vi "serial-read-subVi-SAFEish.vi"(8 "error in":errorcluster, 10 "state":string="init", 11 "VISA resource name":refnum<visa-resource-name>="COM22") -> (0 "error out":errorcluster, 1 "read buffer out":string, 2 "all-sensor-data":T4 {"CD4"."CO2 (ppm)" format="%.2f"; "CD3"."CO2 (ppm)" format="%.2f"; "RHT4"."Humidity (%)" format="%.2f"; "RHT4"."Temp (degC)" format="%.2f"; "RHT5"."Humidity (%)" format="%.2f"; "RHT5"."Temp (degC)" format="%.2f"; "CD2"."Humidity (%)" format="%.2f"; "CD2"."Temp (degC)" format="%.2f"; "CD2"."CO2 (ppm)" format="%.2f"; "RHT3"."Humidity (%)" format="%.2f"; "RHT3"."Temp (degC)" format="%.2f"; "CD6"."CO2 (ppm)" format="%.2f"; "RHT6"."Humidity (%)" format="%.2f"; "RHT6"."Temp (degC)" format="%.2f"; "CD5"."CO2 (ppm)" format="%.2f"; "CD1"."Humidity (%)" format="%.2f"; "CD1"."Temp (degC)" format="%.2f"; "CD1"."CO2 (ppm)" format="%.2f"}, 3 "VISA resource out":refnum<visa-resource-name>)   [LabVIEW 2021]
uses:
  all-sensor-data.ctl
  SCD41.ctl
  STC31.ctl
  SHT41.ctl
  <vilib>/Instr/_visa.llb/VISA Configure Serial Port (Instr).vi
panel:
  out "x > y?":bool
  out "RHT4":T1 {"Humidity (%)" format="%.2f"; "Temp (degC)" format="%.2f"}
  out "RHT3":T1 {"Humidity (%)" format="%.2f"; "Temp (degC)" format="%.2f"}
  out "RHT6":T1 {"Humidity (%)" format="%.2f"; "Temp (degC)" format="%.2f"}
  out "RHT5":T1 {"Humidity (%)" format="%.2f"; "Temp (degC)" format="%.2f"}
  out "CD6":T2 {"CO2 (ppm)" format="%.2f"}
  out "CD5":T2 {"CO2 (ppm)" format="%.2f"}
  out "CD4":T2 {"CO2 (ppm)" format="%.2f"}
  out "CD3":T2 {"CO2 (ppm)" format="%.2f"}
  out "CD2":T3 {"Humidity (%)" format="%.2f"; "Temp (degC)" format="%.2f"; "CO2 (ppm)" format="%.2f"}
  out "CD1":T3 {"Humidity (%)" format="%.2f"; "Temp (degC)" format="%.2f"; "CO2 (ppm)" format="%.2f"}
  out "Num Samples":i32
  out "data string array":string[](array[string])
  out "read buffer":string
  out "Bytes Returned":u32
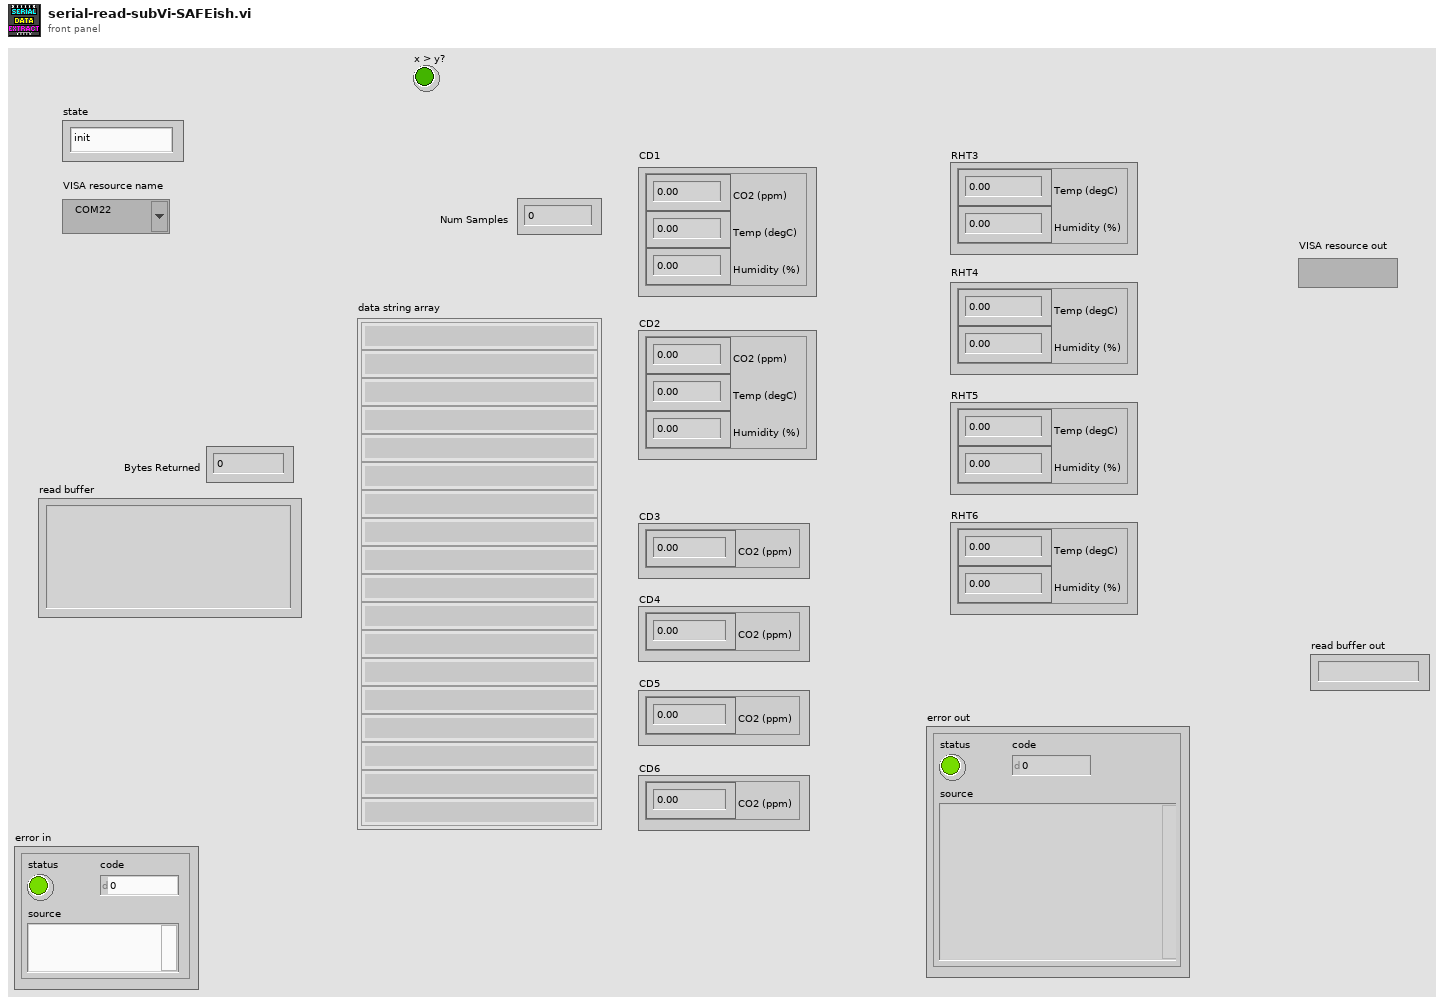
[diagram p1: front panel]
types:
  T1 = typedef "SHT41.ctl" = cluster{"Temp (degC)":dbl, "Humidity (%)":dbl}
  T2 = typedef "STC31.ctl" = cluster{"CO2 (ppm)":dbl}
  T3 = typedef "SCD41.ctl" = cluster{"CO2 (ppm)":dbl, "Temp (degC)":dbl, "Humidity (%)":dbl}
  T4 = typedef "all-sensor-data.ctl" = cluster{"CD1":T3, "CD2":T3, "CD3":T2, "CD4":T2, "CD5":T2, "CD6":T2, "RHT3":T1, "RHT4":T1, "RHT5":T1, "RHT6":T1}
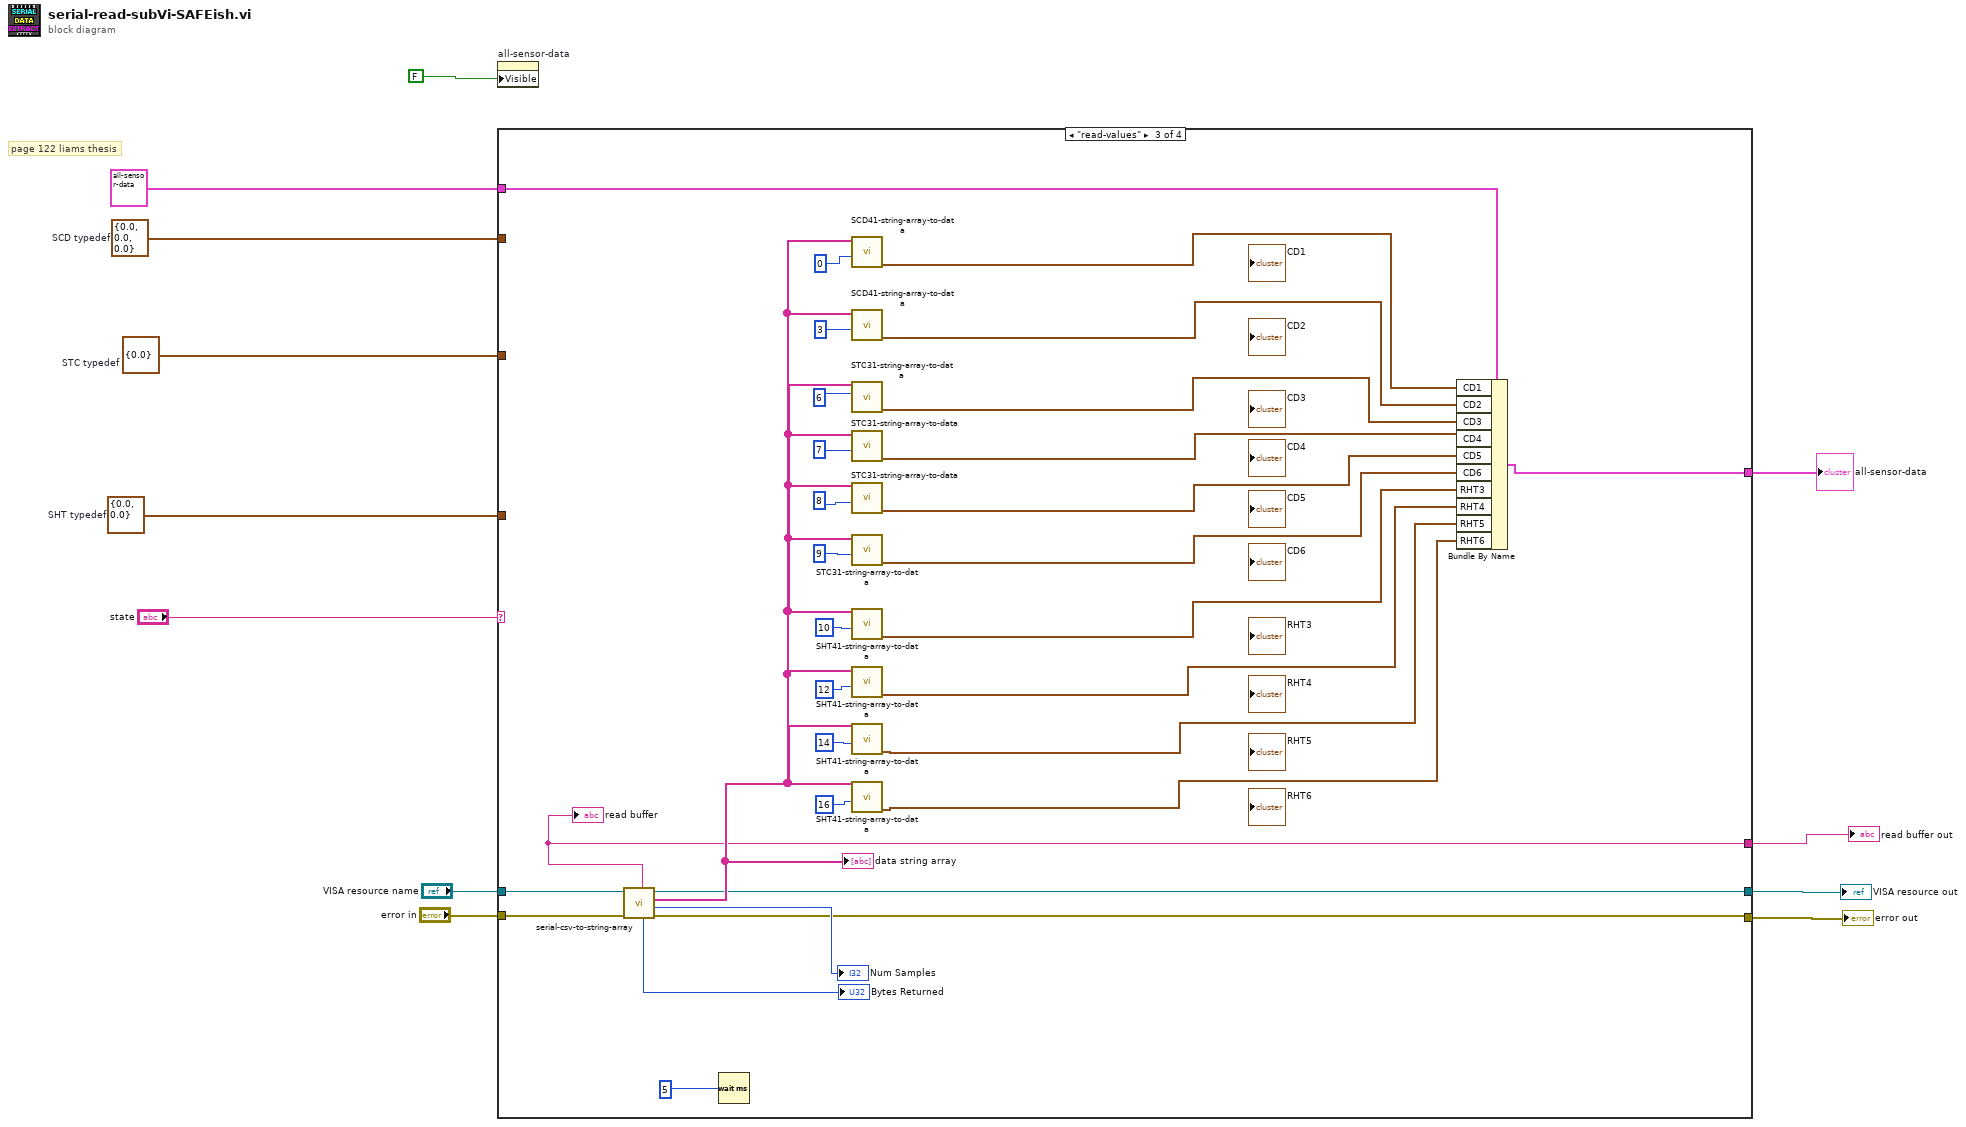
[diagram p0: block diagram]
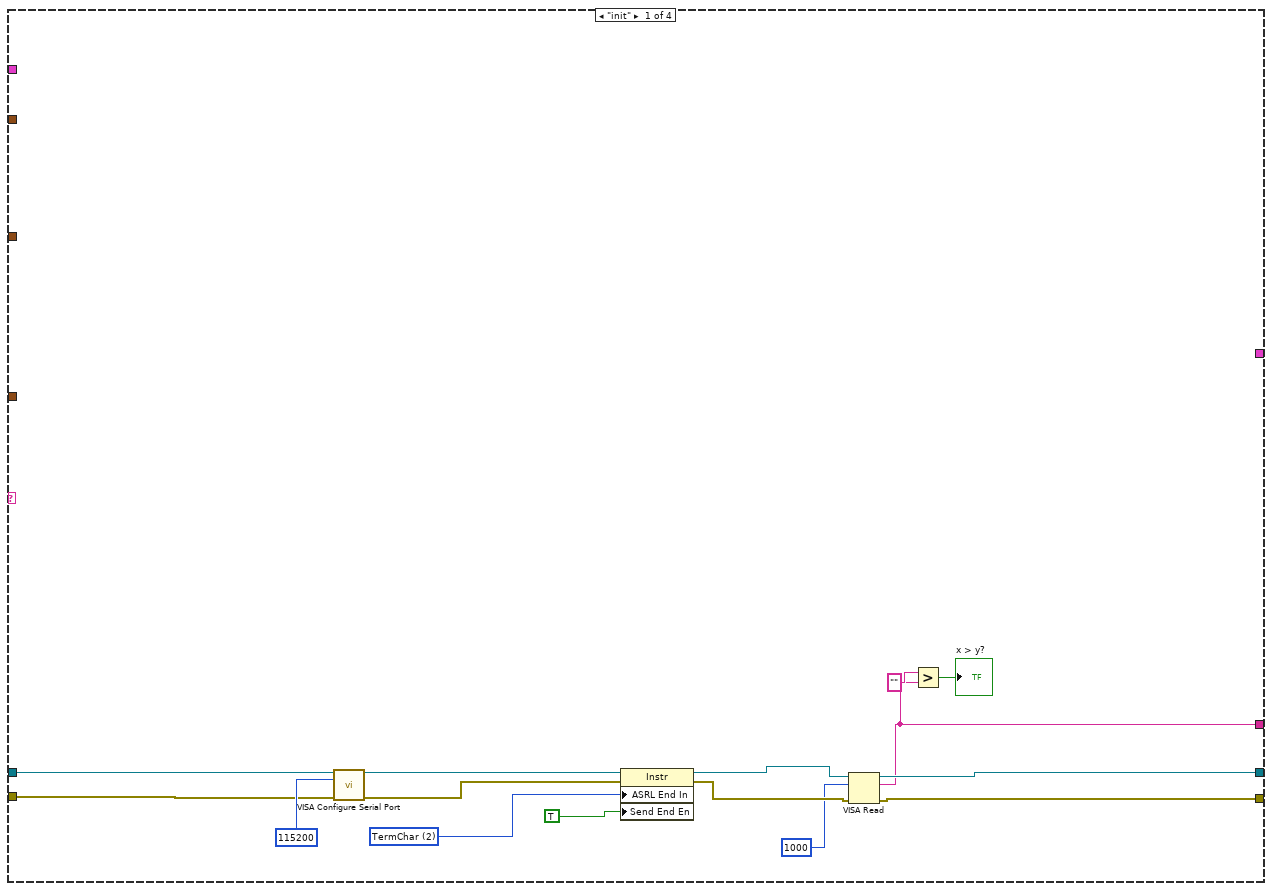
[diagram p2: hidden frame]
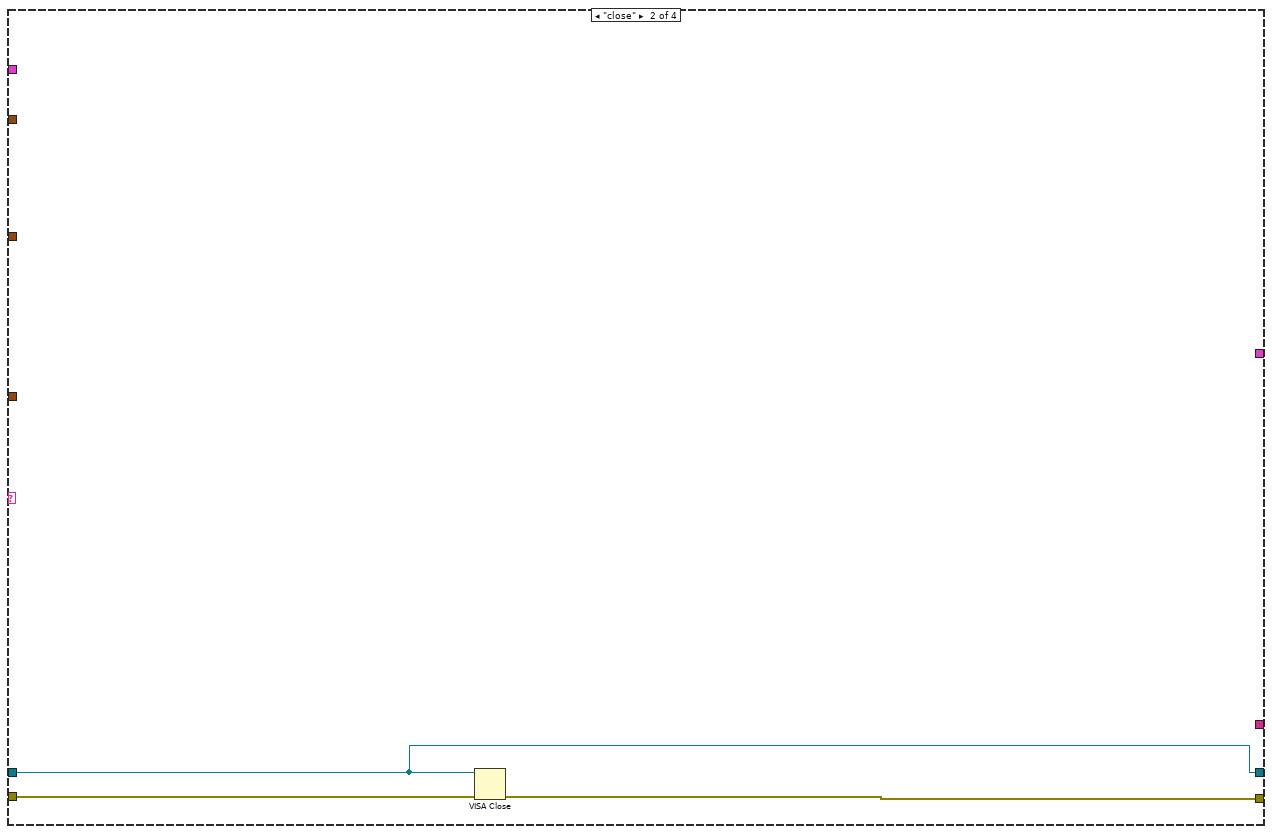
[diagram p3: hidden frame]
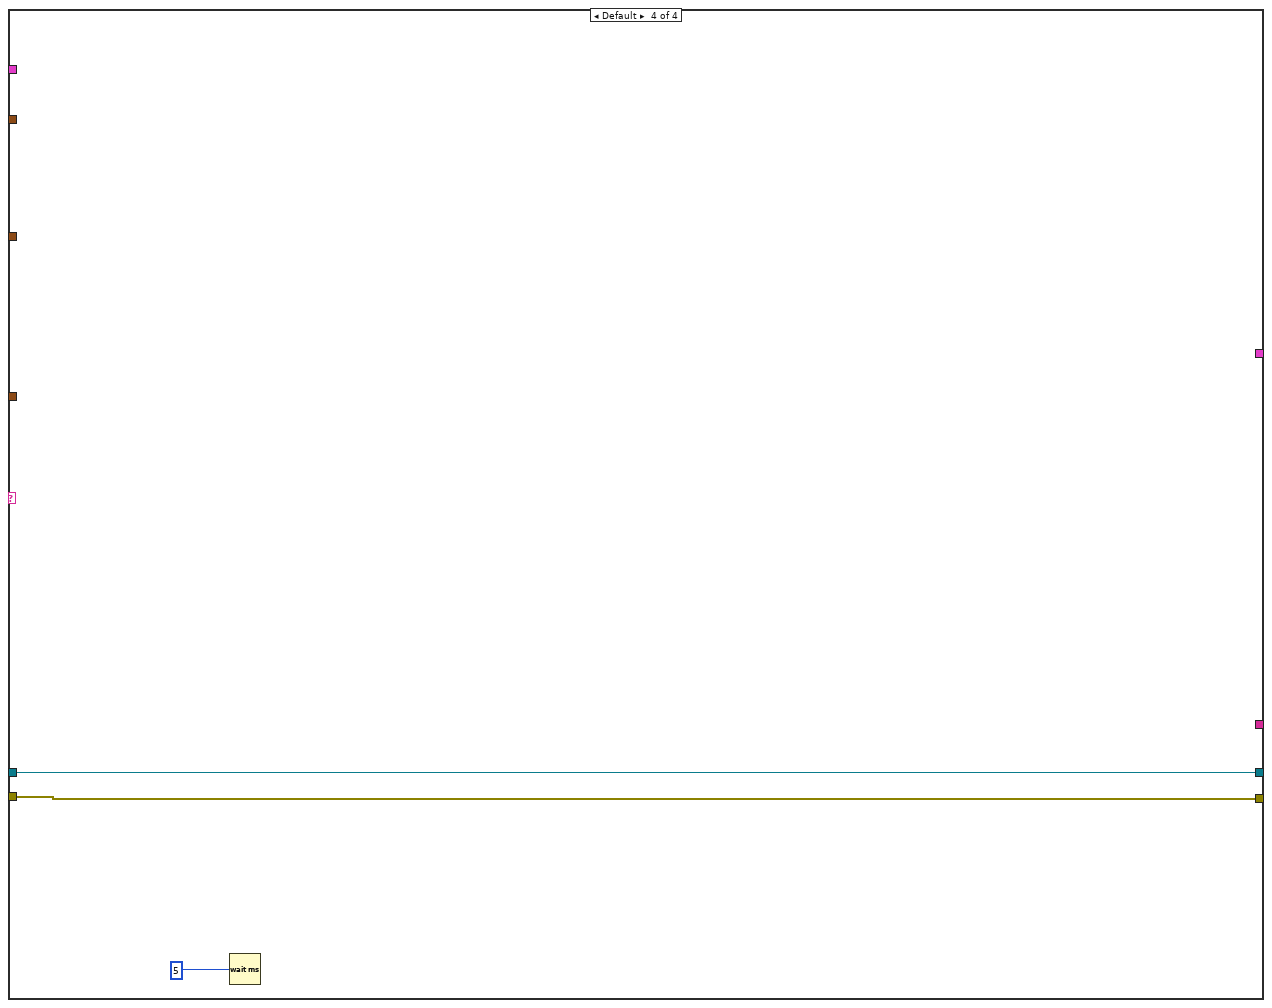
[diagram p4: hidden frame]
diagram:
  w8 = T1 {"Temp (degC)"=0.0, "Humidity (%)"=0.0}  # SHT typedef
  w9 = T2 {"CO2 (ppm)"=0.0}  # STC typedef
  w10 = T3 {"CO2 (ppm)"=0.0, "Temp (degC)"=0.0, "Humidity (%)"=0.0}  # SCD typedef
  # "page 122 liams thesis"
  n1 = property on="all-sensor-data" class="Clust (strict)"("Visible"=FALSE) -> ()  [unwired: 2 in, 2 out]
  n2 = case shown="\"read-values\"" "state" {
    tunnel: "VISA resource name" -> [w22 w28 w49 w63]
    tunnel: w10 -> [_ _ _ _]
    tunnel: w9 -> [_ _ _ _]
    tunnel: w8 -> [_ _ _ _]
    tunnel: T4 {"CD1"={"CO2 (ppm)"=0.0, "Temp (degC)"=0.0, "Humidity (%)"=0.0}, "CD2"={"CO2 (ppm)"=0.0, "Temp (degC)"=0.0, "Humidity (%)"=0.0}, "CD3"={"CO2 (ppm)"=0.0}, "CD4"={"CO2 (ppm)"=0.0}, "CD5"={"CO2 (ppm)"=0.0}, "CD6"={"CO2 (ppm)"=0.0}, "RHT3"={"Temp (degC)"=0.0, "Humidity (%)"=0.0}, "RHT4"={"Temp (degC)"=0.0, "Humidity (%)"=0.0}, "RHT5"={"Temp (degC)"=0.0, "Humidity (%)"=0.0}, "RHT6"={"Temp (degC)"=0.0, "Humidity (%)"=0.0}} ("all-data") -> [_ _ w50 _]
    tunnel: "error in" -> [w21 w30 w48 w62]
    tunnel: [w17 w29 w33 w62] -> w5
    tunnel: [w19 w28 w34 w63] -> w4
    tunnel: [w16 _ w32 _] -> w1
    tunnel: [_ _ w31 _] -> w2
    frame "init" {
      w25 = u16 2 items=["None", "Last Bit", "TermChar"] ("Serial Settings:End Mode for Reads")
      n3 = call-poly "VISA Configure Serial Port"("VISA resource name"=w22, "baud rate (9600)"=u32 115200, "error in (no error)"=w21) -> ("VISA resource name out"=w26:refnum<visa-resource-name>, "error out"=w27:errorcluster)  [unwired: 11 in]
      n4 = property class="Instr"(reference=w26, error in=w27, "ASRL End In"=w25, "Send End En"=TRUE ("Message Based Settings:Send End Enable")) -> (reference out=w20:refnum<visa-resource-name>, error out=w18:errorcluster)
      n5 = VISA Read(VISA resource name=w20, byte count=u32 1000, error in (no error)=w18) -> (VISA resource name out=w19:refnum<visa-resource-name>, read buffer=w16:string, error out=w17:errorcluster)  [unwired: 1 out]
      n6 = Greater?(x=w16, y="") -> (0:→"x > y?":bool)
    }
    frame "close" {
      n7 = VISA Close(VISA resource name=w28, error in (no error)=w30) -> (error out=w29:errorcluster)
    }
    frame "read-values" {
      n8 = call "serial-csv-to-string-array.vi"("error in (no error)"=w48, "VISA Refnum in"=w49) -> ("error out"=w33:errorcluster, "Num Samples Reported"=→"Num Samples":i32, "data string array"=w47:string[], "VISA Refnum out"=w34:refnum<visa-resource-name>, "Bytes Returned"=→"Bytes Returned":u32, "read buffer"=w32:string)  [unwired: 4 in]
      "read buffer" <- w32
      "data string array" <- w47
      n9 = Wait (ms)(milliseconds to wait=u32 5) -> ()  [unwired: 1 out]
      n10 = call "SCD41-string-array-to-data.vi"("Starting Index"=0, "Data In (string array)"=w47) -> ("SCD41: data output"=w46:T3)  [unwired: 6 in, 3 out]
      n11 = call "SCD41-string-array-to-data.vi"("Starting Index"=3, "Data In (string array)"=w47) -> ("SCD41: data output"=w45:T3)  [unwired: 6 in, 3 out]
      n12 = call "STC31-string-array-to-data.vi"("Starting Index"=6 ("index"), "Data In (string array)"=w47) -> ("STC31: data output"=w44:T2)  [unwired: 7 in, 2 out]
      n13 = call "STC31-string-array-to-data.vi"("Starting Index"=7, "Data In (string array)"=w47) -> ("STC31: data output"=w43:T2)  [unwired: 7 in, 2 out]
      n14 = call "STC31-string-array-to-data.vi"("Starting Index"=8, "Data In (string array)"=w47) -> ("STC31: data output"=w42:T2)  [unwired: 7 in, 2 out]
      n15 = call "STC31-string-array-to-data.vi"("Starting Index"=9, "Data In (string array)"=w47) -> ("STC31: data output"=w41:T2)  [unwired: 7 in, 2 out]
      n16 = call "SHT41-string-array-to-data.vi"("Starting Index"=10, "Data In (string array)"=w47) -> ("SHT41: data output"=w40:T1)  [unwired: 7 in, 2 out]
      n17 = call "SHT41-string-array-to-data.vi"("Starting Index"=12, "Data In (string array)"=w47) -> ("SHT41: data output"=w39:T1)  [unwired: 7 in, 2 out]
      n18 = call "SHT41-string-array-to-data.vi"("Starting Index"=14, "Data In (string array)"=w47) -> ("SHT41: data output"=w38:T1)  [unwired: 7 in, 2 out]
      n19 = call "SHT41-string-array-to-data.vi"("Starting Index"=16, "Data In (string array)"=w47) -> ("SHT41: data output"=w37:T1)  [unwired: 7 in, 2 out]
      n20 = Bundle By Name(cluster=w50, "CD1"=w46, "CD2"=w45, "CD3"=w44, "CD4"=w43, "CD5"=w42, "CD6"=w41, "RHT3"=w40, "RHT4"=w39, "RHT5"=w38, "RHT6"=w37) -> (w31:T4)
    }
    frame Default {
      n21 = Wait (ms)(milliseconds to wait=u32 5) -> ()  [unwired: 1 out]
    }
  }
  "error out" <- w5
  "VISA resource out" <- w4
  "all-sensor-data" <- w2
  "read buffer out" <- w1
